vi "Network-Write Length-Prefixed String.vi"(0 "connection ID":refnum<k5>, 7 "String":string, 9 "timeout (ms)":i32=5000, 11 "error in (no error)":errorcluster) -> (4 "connection ID out":refnum<k5>, 15 "error out":errorcluster)   [LabVIEW 2020]
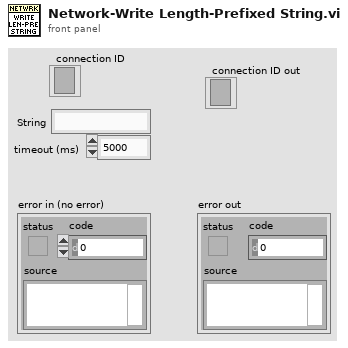
[diagram p1: front panel]
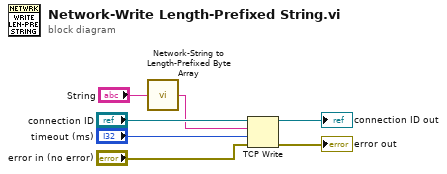
[diagram p0: block diagram]
diagram:
  n1 = call "Network-String to Length-Prefixed Byte Array.vi"("String"="String") -> ("String"=w3:string)  [unwired: 14 in]
  n2 = TCP Write(connection ID="connection ID", data in=w3, error in (no error)="error in (no error)", 9:"timeout (ms)") -> (connection ID out=→"connection ID out":refnum<k5>, error out=→"error out":errorcluster)  [unwired: 1 out]
